vi "Find All Writers of Data.vi"(8 "error in (no error)":errorcluster, 10 "Full Element Name":string[](array[string]), 11 "JKI SM in":refnum<class "JKI SM.lvclass">) -> (0 "error out":errorcluster, 1 "InPlaceClusterNode":refnum<vi>[](array[refnum]), 2 "NamedBundlers":refnum<vi>[](array[refnum]), 3 "JKI SM out":refnum<class "JKI SM.lvclass">)   [LabVIEW 2013, in "JKI State Machine API.lvlib" / "JKI SM.lvclass"]
uses:
  JKI SM.lvclass
  <vilib>/Utility/traverseref.llb/TRef TravTarget.ctl
  JKI SM.lvclass/JKI SM.ctl
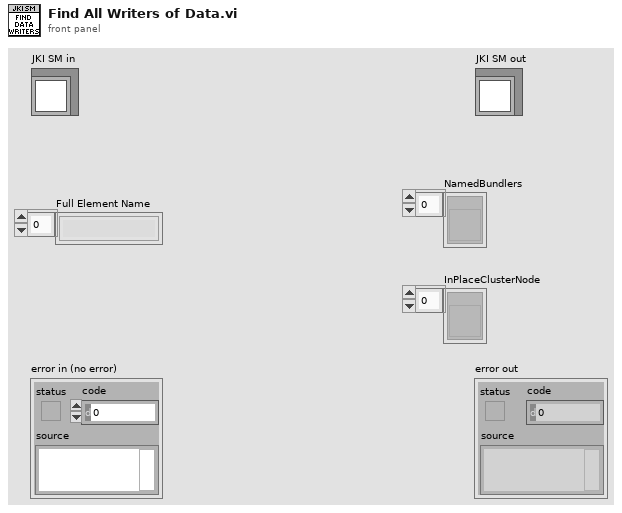
[diagram p1: front panel]
types:
  T1 = typedef "TRef TravTarget.ctl" = enum16{"FP", "BD", "Other"}
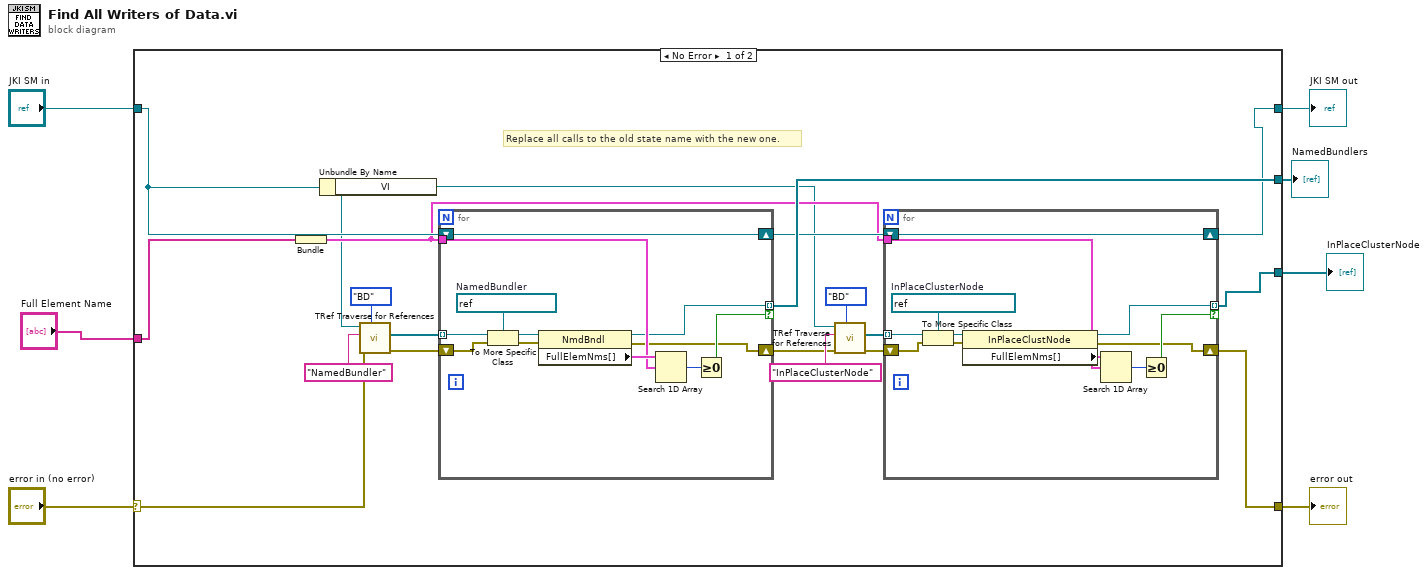
[diagram p0: block diagram]
diagram:
  n1 = case shown="No Error" "error in (no error)" {
    selector: "error in (no error)" -> [w20 w52]
    tunnel: [w11 w52] -> w6
    tunnel: [w9 w51] -> w4
    tunnel: "JKI SM in" -> [w21 w51]
    tunnel: "Full Element Name" -> [w26 _]
    tunnel: [w19 _] -> w2
    tunnel: [w10 _] -> w1
    frame No Error {
      # "Replace all calls to the old state name with the new one."
      n2 = Bundle("Full Element Name"=w26) -> (w17:cluster{"Full Element Name":string[]})  [unwired: 1 in]
      n3 = Unbundle By Name(w21) -> ("VI"=w8:refnum<vi>)
      n4 = call <vilib>:"TRef Traverse for References.vi"("Traverse Target"=TRef_TravTarget."BD", "error in (no error)"=w20, "Class Name"="NamedBundler", "VI Refnum"=w8) -> ("error out"=w22:errorcluster, "References"=w23:refnum<vi>[])  [unwired: 1 in, 5 out]
      n5 = for {
        tunnel: w23 -> [w50] mode=indexing
        tunnel: w17 -> [w44]
        shift-right: [w46] -> w18
        shift-left: w21 -> [w46]
        shift-right: [w40] -> w14
        shift-left: w22 -> [w48]
        tunnel: [w41] -> w19 mode=indexing if=w42
        w39 = refnum<vi> refnum  # NamedBundler
        n6 = To More Specific Class(target class=w39, reference=w50, error in=w48) -> (specific class reference=w49:refnum<vi>, error out=w47:errorcluster)
        n7 = property class="NmdBndl"(reference=w49, error in=w47) -> (reference out=w41:refnum<vi>, error out=w40:errorcluster, "FullElemNms[]"=w45:cluster{string[]}[])
        n8 = Search 1D Array(1D array=w45, element=w44) -> (index of element=w43:i32)  [unwired: 1 in]
        n9 = Greater Or Equal To 0?(x=w43) -> (x >= 0?=w42:bool)
      }
      n10 = call <vilib>:"TRef Traverse for References.vi"("Traverse Target"=TRef_TravTarget."BD", "error in (no error)"=w14, "Class Name"="InPlaceClusterNode", "VI Refnum"=w8) -> ("error out"=w13:errorcluster, "References"=w12:refnum<vi>[])  [unwired: 1 in, 5 out]
      n11 = for {
        tunnel: w12 -> [w38] mode=indexing
        tunnel: w17 -> [w32]
        shift-right: [w34] -> w9
        shift-left: w18 -> [w34]
        shift-right: [w28] -> w11
        shift-left: w13 -> [w36]
        tunnel: [w29] -> w10 mode=indexing if=w30
        w27 = refnum<vi> refnum  # InPlaceClusterNode
        n12 = To More Specific Class(target class=w27, reference=w38, error in=w36) -> (specific class reference=w37:refnum<vi>, error out=w35:errorcluster)
        n13 = property class="InPlaceClustNode"(reference=w37, error in=w35) -> (reference out=w29:refnum<vi>, error out=w28:errorcluster, "FullElemNms[]"=w33:cluster{string[]}[])
        n14 = Search 1D Array(1D array=w33, element=w32) -> (index of element=w31:i32)  [unwired: 1 in]
        n15 = Greater Or Equal To 0?(x=w31) -> (x >= 0?=w30:bool)
      }
    }
    frame Error {
    }
  }
  "error out" <- w6
  "JKI SM out" <- w4
  "NamedBundlers" <- w2
  "InPlaceClusterNode" <- w1
